vi "Stop Core.vi"(10 "final error code":i32, 11 "MainController in":refnum<class "MainController.lvclass">) -> (3 "MainController out":refnum<class "MainController.lvclass">)   [LabVIEW 2012, in "Win8uiFramework.lvlib" / "MainController.lvclass"]
doc: "(<B>Filename</B>: Actor Framework.lvlib:Actor.lvclass:Stop Core.vi)\n\nDefines what the actor does before it stops. Use the <B>final error code</B> input to determine whether the actor shut down in response to an error.\n\nBy default, this method does nothing. A descendant class may override it to define behavior, such as shutting down any processes the actor initiated in its override of the Actor Core method."
uses:
  MainController.lvclass
  MainController.lvclass/MainController.ctl
  ViewableActor.lvclass
  <vilib>/ActorFramework/Message Enqueuer/Message Enqueuer.lvclass/Message Enqueuer.ctl
  Read AppBar Enqueuer.vi
  Read Charm Enqueuer.vi
  Read MainPane Enqueuer.vi
  <vilib>/ActorFramework/Message Enqueuer/Enqueue.vi
  <vilib>/ActorFramework/Message Priority Queue/Priority Enqueue.vi
  <vilib>/ActorFramework/Message Enqueuer/Message Enqueuer.lvclass
  <vilib>/ActorFramework/Stop Msg/Stop Msg.lvclass
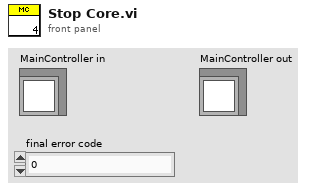
[diagram p1: front panel]
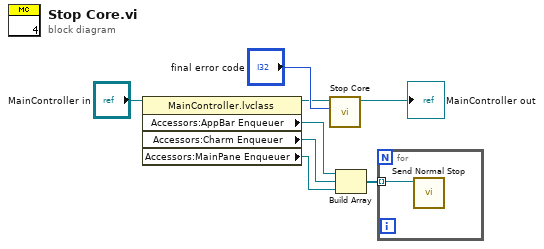
[diagram p0: block diagram]
diagram:
  n1 = property class="MainController.lvclass"(reference="MainController in") -> (reference out=w5:refnum<class "MainController.lvclass">, "Accessors:AppBar Enqueuer"=w3:refnum<class "Message Enqueuer.lvclass">, "Accessors:Charm Enqueuer"=w2:refnum<class "Message Enqueuer.lvclass">, "Accessors:MainPane Enqueuer"=w1:refnum<class "Message Enqueuer.lvclass">)  [unwired: 1 in, 1 out]
  n2 = call-parent "Stop Core.vi"("final error code"="final error code", "ViewableActor in"=w5) -> ("ViewableActor out"=→"MainController out":refnum<class "MainController.lvclass">)  [unwired: 9 in]
  n3 = Build Array(w3, w2, w1) -> (w4:refnum<class "Message Enqueuer.lvclass">[])
  n4 = for {
    tunnel: w4 -> [w9] mode=indexing
    n5 = call <vilib>:"Send Normal Stop.vi"("Message Enqueuer"=w9) -> ()  [unwired: 10 in, 1 out]
  }
